vi "Deadband.vi"(10 "Deadband":dbl=0.1 format="%#_13g", 11 "Input":dbl) -> (3 "Output":dbl)   [LabVIEW 2019]
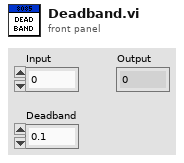
[diagram p1: front panel]
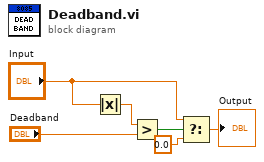
[diagram p0: block diagram]
diagram:
  n1 = Absolute Value(x="Input") -> (abs(x)=w2:dbl)
  n2 = Greater?(x=w2, y="Deadband") -> (0:w1:bool)
  n3 = Select(t="Input", s=w1, f=0.0) -> (s? t:f=→"Output":dbl)
